vi "citTemplate.sendAckNotifier.vi"(0 "notification data":string, 2 "notifierHandle in":T2, 11 "error in":errorcluster) -> ()   [LabVIEW 2019, in "Tools.lvlib"]
uses:
  Tools.lvlib
  citTemplate.notifierHandle.ctl
  citTemplate.notifierData.ctl
panel:
  in  "notifierData":T1
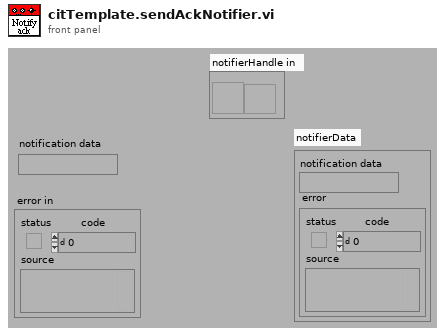
[diagram p1: front panel]
types:
  T1 = typedef "Tools.lvlib/citTemplate.notifierData.ctl" = cluster{"notification data":string, "error":errorcluster}
  T2 = typedef "Tools.lvlib/citTemplate.notifierHandle.ctl" = refnum<notifier>
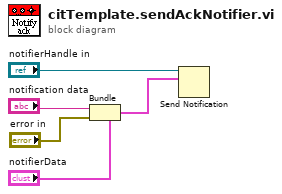
[diagram p0: block diagram]
diagram:
  n1 = Bundle(cluster="notifierData", "notification data"="notification data", "error"="error in") -> (w4:T1)
  n2 = Send Notification(notification=w4, notifier="notifierHandle in") -> ()  [unwired: 1 in, 2 out]
